vi "水样测试.vi"(11 "数据标记表":string(combo)="N") -> ()   [LabVIEW 2016, in "斯坦道多参数.lvlib"]
panel:
  out "运行状态":u16(ring) items=["空闲", "水样测试", "标样核查"]
  out "多参数运行日志":string
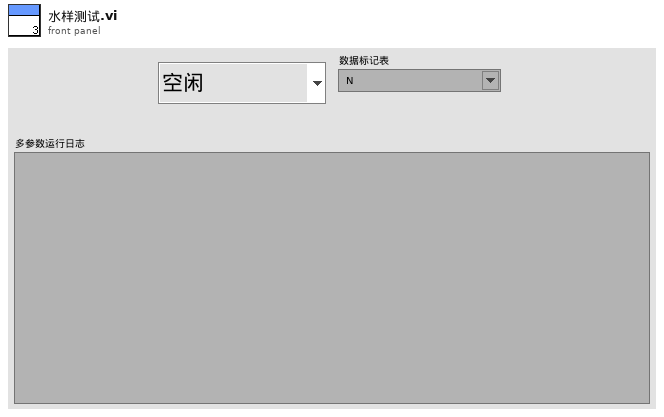
[diagram p1: front panel]
types:
  T1 = typedef "集成多参数单参数字段定义.ctl" = cluster{"时间":timestamp, "测量模式":string, "数据类型":string, "检测值":sgl, "单位":string, "数据标识":string, "信号值":sgl, "标样参考值":sgl, "因子编码":string, "探头温度":sgl, "LastTime":timestamp}
  T2 = cluster{"水温":bool, "pH":bool, "DO":bool, "DOper":bool, "电导率":bool, "ORP":bool, "浊度":bool, "叶绿素a":bool, "藻密度":bool, "COD":bool, "DO2":bool, "DOper":bool}
  T3 = cluster{"水样数据时间":timestamp, "水温":dbl, "pH":dbl, "DO":dbl, "DOper":dbl, "电导率":dbl, "ORP":dbl, "浊度":dbl, "叶绿素a":dbl, "藻密度":dbl, "COD":dbl, "DO2":dbl, "DO2per":dbl}
  T4 = cluster{"ph":bool, "DO":bool, "Cond":bool, "Turb":bool, "叶绿素a":bool, "藻密度":bool, "ORP":bool, "cod":bool, "DO2":bool}
  T5 = cluster{"温度测量值":sgl, "测量值":sgl, "温度偏移修正值":sgl, "信号值":sgl, "数据标识":string}
  T6 = cluster{"CH":u16, "监测值":dbl, "信号值":sgl, "数据标识":string}
  T7 = cluster{"温度测量值":sgl, "DO%":sgl, "DOmg/L":sgl, "温度偏移修正值":sgl, "数据标识mg/L":string, "数据标识%":string}
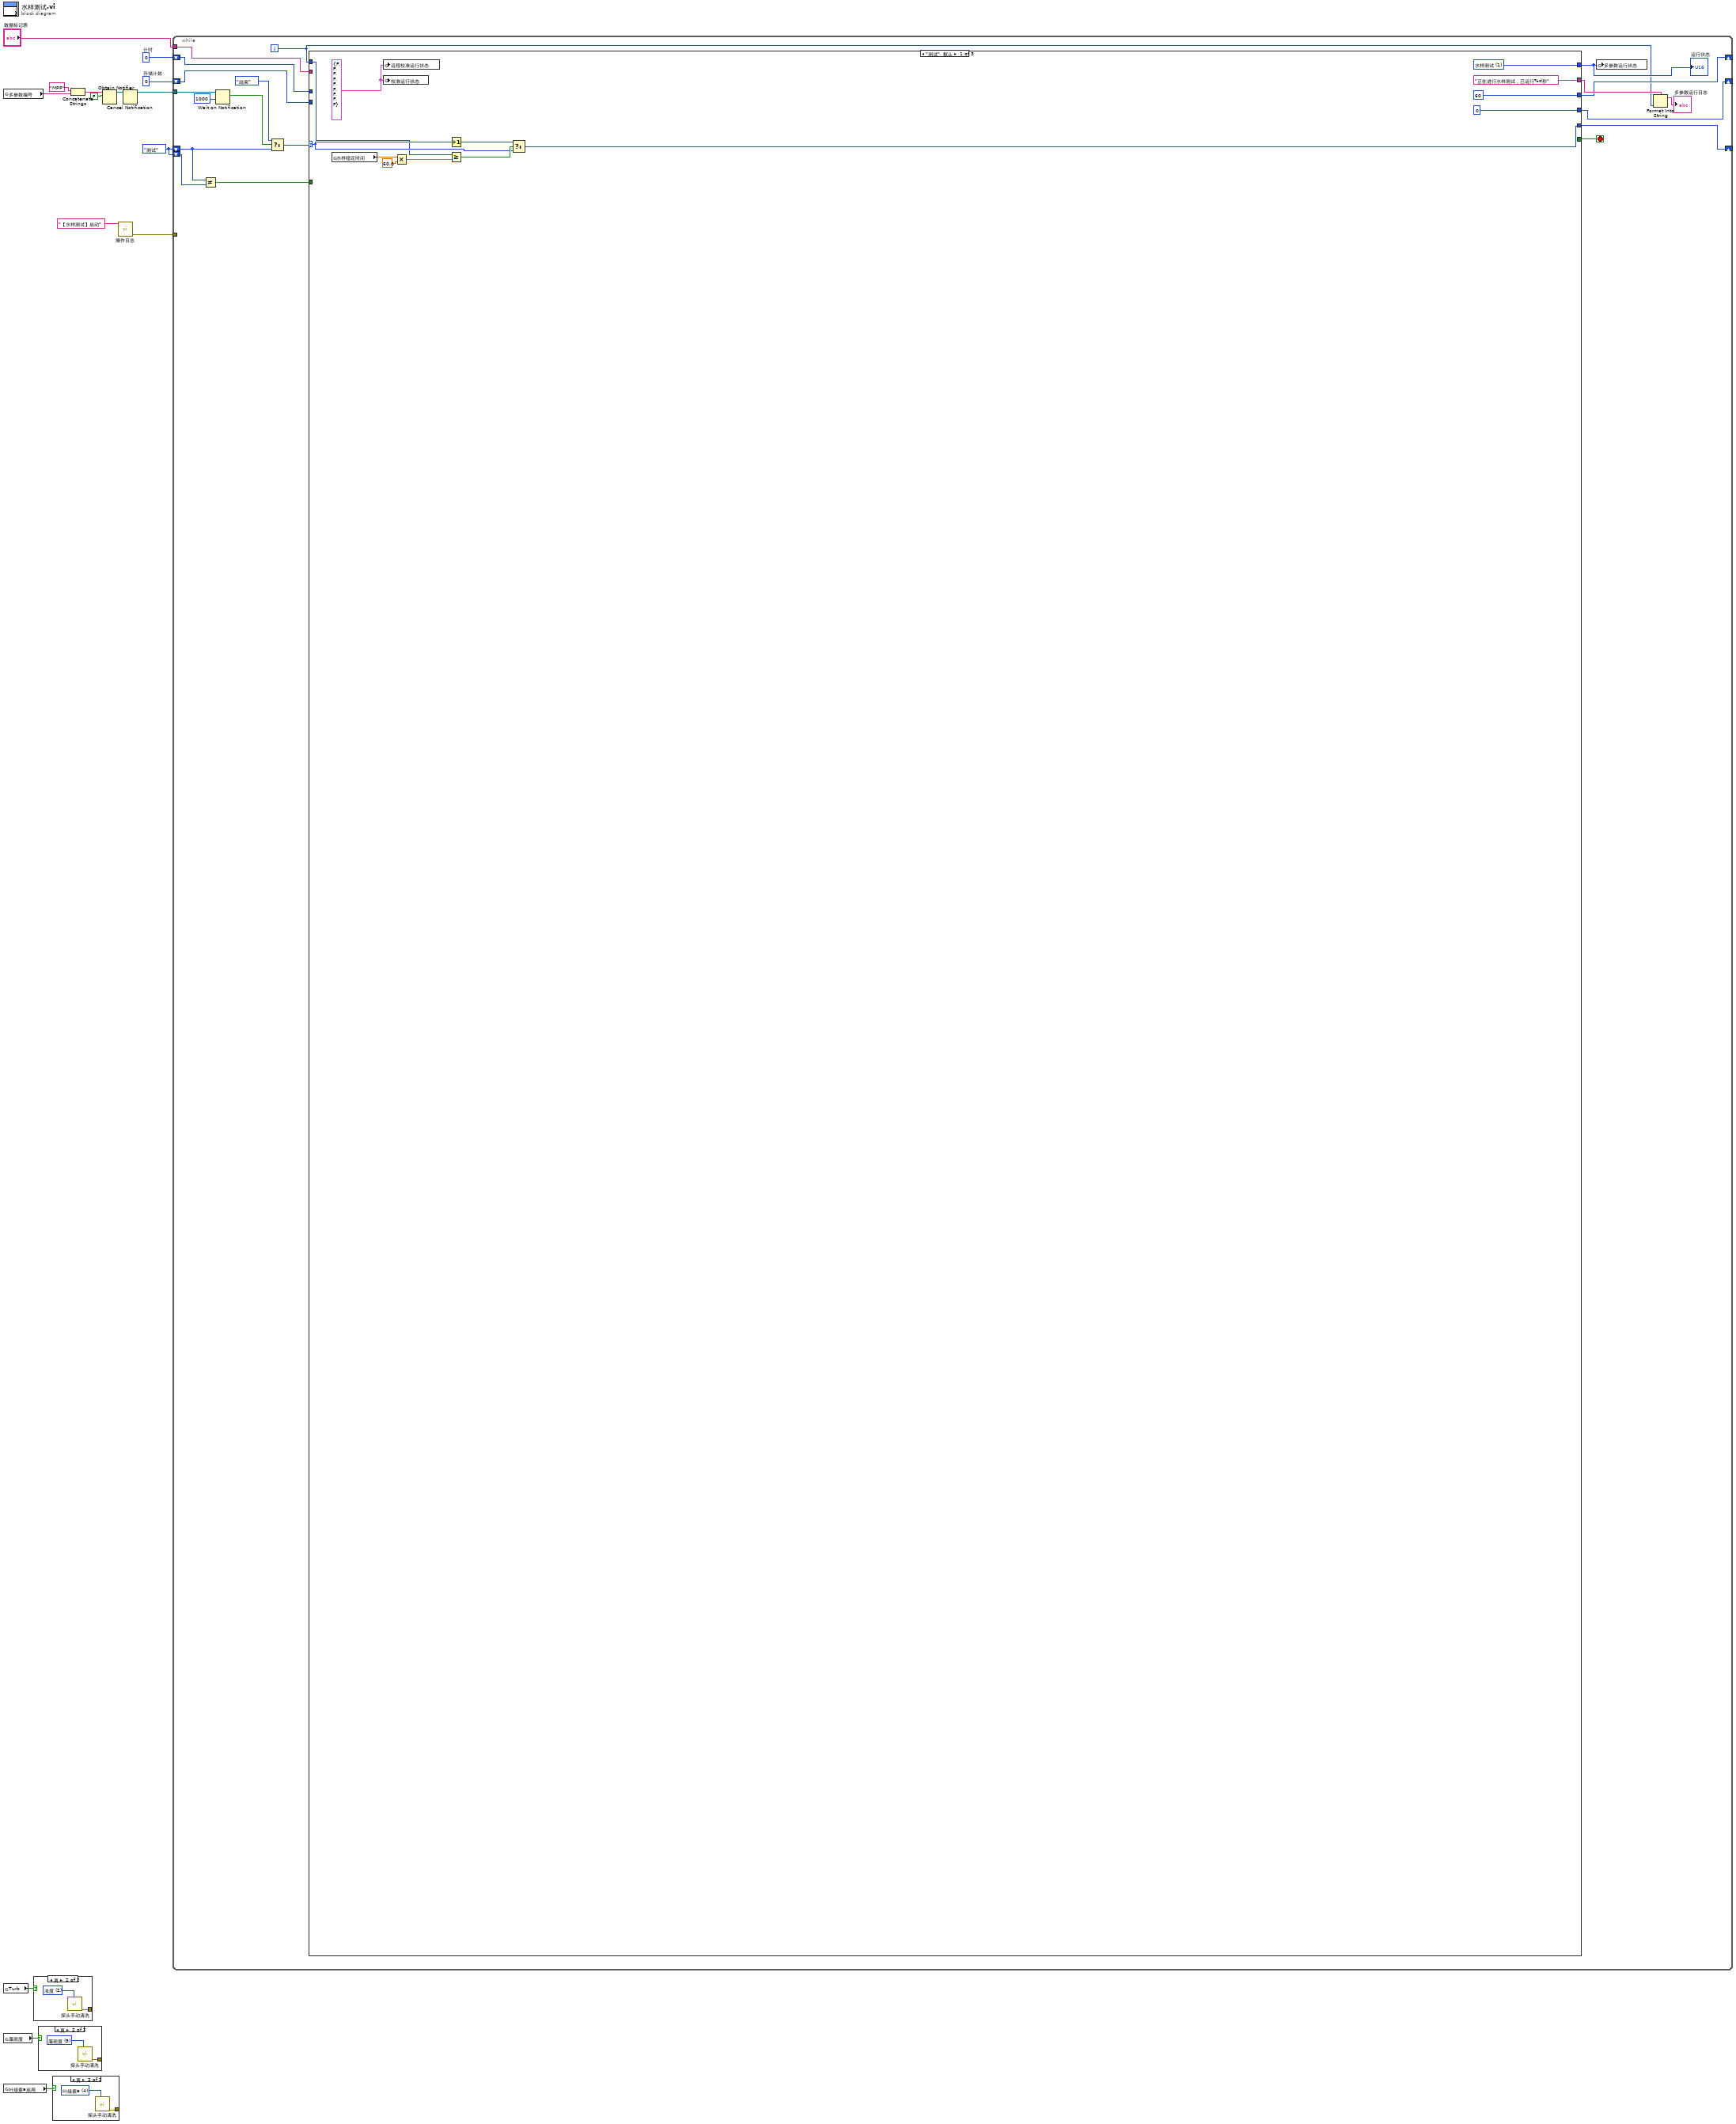
[diagram p0: block diagram]
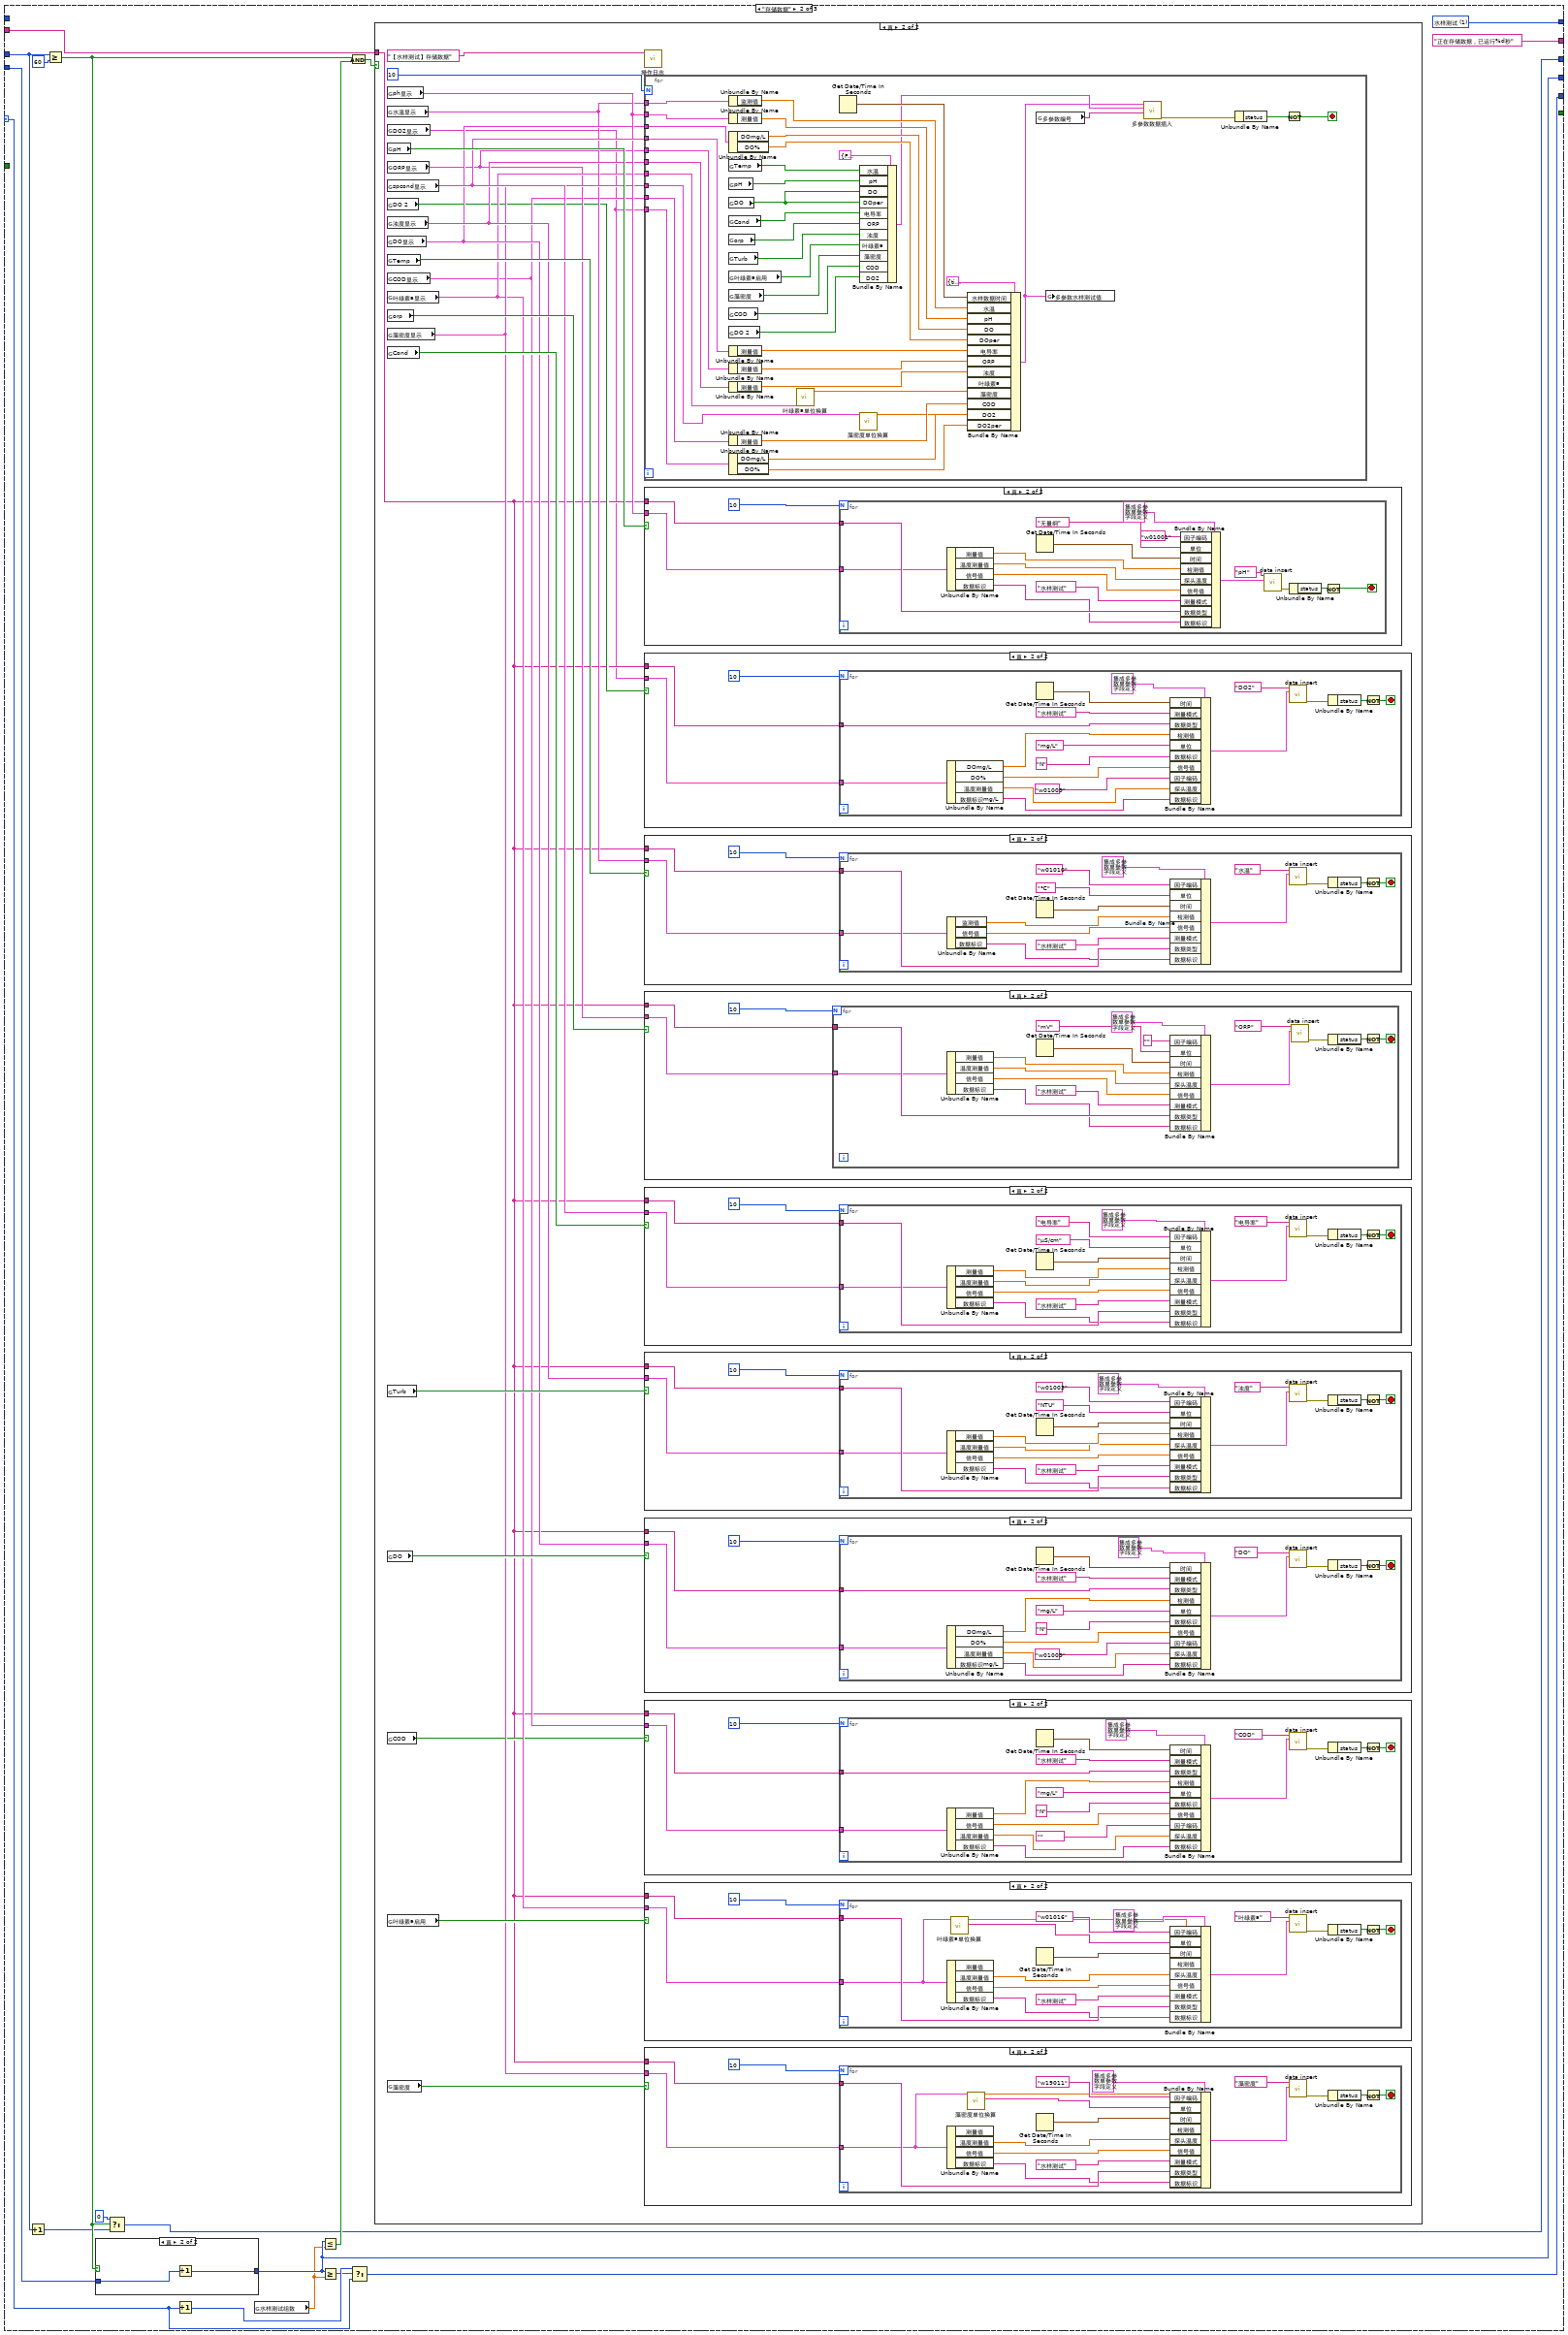
[diagram p5: hidden frame]
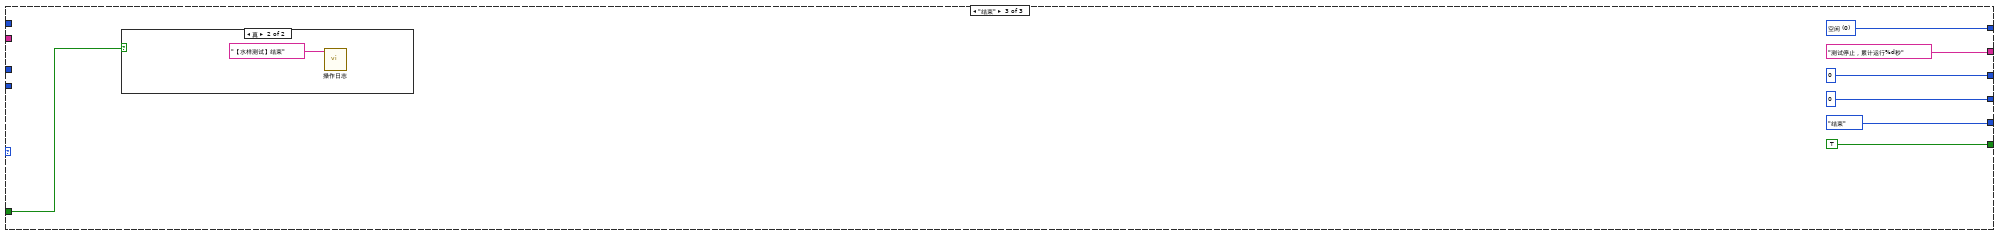
[diagram p18: hidden frame]
diagram:
  w7 = 0  # 存储计数
  w8 = 0  # 计时
  w3 = enum16{"测试", "存储数据", "结束"}."测试" ("枚举")
  n1 = global read "多参数全局变量.vi" "多参数编号"() -> (w9:string)
  n2 = global read "断电保存变量.vi" "Turb"() -> (w6:bool)
  n3 = global read "断电保存变量.vi" "藻密度"() -> (w4:bool)
  n4 = global read "断电保存变量.vi" "叶绿素a启用"() -> (w5:bool)
  n5 = case shown="真" w6 {
    tunnel: [_ w16] -> _
    frame False {
    }
    frame True {
      w17 = u16 2 items=["pH", "DO", "浊度", "电导率", "叶绿素a", "藻密度", "ORP", "DO2"] ("校准参数")
      n6 = call "探头手动清洗.vi"("校准参数"=w17) -> ("error out"=w16:errorcluster)  [unwired: 10 in]
    }
  }
  n7 = case shown="真" w4 {
    tunnel: [_ w18] -> _
    frame False {
    }
    frame True {
      w19 = u16 5 items=["pH", "DO", "浊度", "电导率", "叶绿素a", "藻密度", "ORP", "DO2"] ("校准参数")
      n8 = call "探头手动清洗.vi"("校准参数"=w19) -> ("error out"=w18:errorcluster)  [unwired: 10 in]
    }
  }
  n9 = case shown="真" w5 {
    tunnel: [_ w20] -> _
    frame False {
    }
    frame True {
      w21 = u16 4 items=["pH", "DO", "浊度", "电导率", "叶绿素a", "藻密度", "ORP", "DO2"] ("校准参数")
      n10 = call "探头手动清洗.vi"("校准参数"=w21) -> ("error out"=w20:errorcluster)  [unwired: 10 in]
    }
  }
  n11 = Concatenate Strings("MPP" ("名称（未命名）"), w9) -> (w10:string)
  n12 = Obtain Notifier(name (unnamed)=w10, notification data type=FALSE) -> (notifier out=w13:refnum<notifier>)  [unwired: 2 in, 2 out]
  n13 = call "操作日志.vi"("日志信息"="【水样测试】启动") -> ("error out"=w1:errorcluster)  [unwired: 10 in]
  n14 = Cancel Notification(0:w13) -> (8:w12:refnum<notifier>)  [unwired: 1 in, 2 out]
  n15 = while {
    shift-right: [w26] -> _
    shift-left: w3 -> [w24]
    tunnel: w12 -> [w37]
    tunnel: "数据标记表" -> [w32]
    shift-right: [w28] -> _
    shift-left: w8 -> [w30]
    shift-right: [w27] -> _
    shift-left: w7 -> [w29]
    shift-left: w3 -> [w23]
    tunnel: w1 -> [_]
    i -> [w25]
    stop <- w40 stop-if-true
    n16 = Not Equal?(x=w24, y=w23) -> (x != y?=w22:bool)
    n17 = Wait on Notification(notifier=w37, timeout in ms (-1)=1000 ("超时毫秒(-1)")) -> (notification=w35:bool)  [unwired: 2 in, 3 out]
    n18 = Select(t=enum16{"测试", "存储数据", "结束"}."结束" ("枚举"), s=w35, f=w24) -> (s? t:f=w33:enum16{"测试", "存储数据", "结束"})
    n19 = case shown="\"测试\", 默认" w33 {
      selector: w33 -> [w47 w61 _]
      tunnel: [_ _ TRUE] -> w40
      tunnel: ["正在进行水样测试，已运行%d秒" ("格式字符串") "正在存储数据，已运行%d秒" ("格式字符串") "测试停止，累计运行%d秒" ("格式字符串")] -> w39
      tunnel: [w52 w66 w335] -> w31
      tunnel: w32 -> [_ w71 _]
      tunnel: w30 -> [_ w69 _]
      tunnel: w29 -> [_ w70 _]
      tunnel: [60 w54 0] -> w28
      tunnel: [0 w60 0] -> w27
      tunnel: [w45 w64 enum16{"测试", "存储数据", "结束"}."结束" ("枚举")] -> w26
      tunnel: w25 -> [w41 _ _]
      tunnel: w22 -> [_ _ w331]
      frame "测试", Default {
        w42 = T4 {"ph"=FALSE, "DO"=FALSE, "Cond"=FALSE, "Turb"=FALSE, "叶绿素a"=FALSE, "藻密度"=FALSE, "ORP"=FALSE, "cod"=FALSE, "DO2"=FALSE} ("远程校准运行状态")
        w52 = u16 1 items=["空闲", "水样测试", "标样核查"] ("多参数运行状态")
        n20 = global read "断电保存变量.vi" "水样稳定时间"() -> (w51:dbl)
        n21 = global write "多参数全局变量.vi" "远程校准运行状态"(w42) -> ()
        n22 = global write "多参数全局变量.vi" "校准运行状态"(w42) -> ()
        n23 = Multiply(x=w51, y=60.0) -> (x*y=w49:dbl)
        n24 = Increment(x=w47) -> (x+1=w46:enum16{"测试", "存储数据", "结束"})
        n25 = Greater Or Equal?(x=w41, y=w49) -> (x >= y?=w48:bool)
        n26 = Select(t=w46, s=w48, f=w47) -> (s? t:f=w45:enum16{"测试", "存储数据", "结束"})
      }
      frame "存储数据" {
        w66 = u16 1 items=["空闲", "水样测试", "标样核查"] ("多参数运行状态")
        n27 = Increment(x=w69) -> (x+1=w56:i32)
        n28 = Greater Or Equal?(x=w69, y=60) -> (x >= y?=w57:bool)
        n29 = case shown="真" w57 {
          tunnel: w70 -> [w72 w74]
          tunnel: [w72 w73] -> w60
          frame False {
          }
          frame True {
            n30 = Increment(x=w74) -> (x+1=w73:i32)
          }
        }
        n31 = Select(t=0, s=w57, f=w56) -> (s? t:f=w54:i32)
        n32 = Increment(x=w61) -> (x+1=w62:enum16{"测试", "存储数据", "结束"})
        n33 = global read "断电保存变量.vi" "水样测试组数"() -> (w59:dbl)
        n34 = Less Or Equal?(x=w60, y=w59) -> (x <= y?=w65:bool)
        n35 = Greater Or Equal?(x=w60, y=w59) -> (x >= y?=w58:bool)
        n36 = And(x=w57, y=w65) -> (x .and. y?=w63:bool)
        n37 = Select(t=w62, s=w58, f=w61) -> (s? t:f=w64:enum16{"测试", "存储数据", "结束"})
        n38 = case shown="真" w63 {
          tunnel: w71 -> [_ w76]
          frame False {
          }
          frame True {
            n39 = global read "多参数全局变量.vi" "ph显示"() -> (w87:T5)
            n40 = global read "多参数全局变量.vi" "水温显示"() -> (w83:T6)
            n41 = global read "多参数全局变量.vi" "DO2显示"() -> (w75:T7)
            n42 = global read "断电保存变量.vi" "pH"() -> (w93:bool)
            n43 = global read "多参数全局变量.vi" "ORP显示"() -> (w81:T5)
            n44 = global read "多参数全局变量.vi" "spcond显示"() -> (w88:T5)
            n45 = global read "断电保存变量.vi" "DO 2"() -> (w77:bool)
            n46 = global read "多参数全局变量.vi" "浊度显示"() -> (w86:T5)
            n47 = global read "多参数全局变量.vi" "DO显示"() -> (w85:T7)
            n48 = global read "断电保存变量.vi" "Temp"() -> (w92:bool)
            n49 = global read "多参数全局变量.vi" "COD显示"() -> (w79:T5)
            n50 = global read "多参数全局变量.vi" "叶绿素a显示"() -> (w82:T5)
            n51 = global read "断电保存变量.vi" "orp"() -> (w90:bool)
            n52 = global read "多参数全局变量.vi" "藻密度显示"() -> (w84:T5)
            n53 = global read "断电保存变量.vi" "Cond"() -> (w95:bool)
            n54 = global read "断电保存变量.vi" "Turb"() -> (w96:bool)
            n55 = global read "断电保存变量.vi" "DO"() -> (w94:bool)
            n56 = global read "断电保存变量.vi" "COD"() -> (w78:bool)
            n57 = global read "断电保存变量.vi" "叶绿素a启用"() -> (w97:bool)
            n58 = global read "断电保存变量.vi" "藻密度"() -> (w91:bool)
            n59 = call "操作日志.vi"("日志信息"="【水样测试】存储数据") -> ()  [unwired: 10 in, 1 out]
            n60 = for {
              N: 10 -> [_]
              tunnel: w83 -> [w158]
              tunnel: w87 -> [w157]
              tunnel: w85 -> [w156]
              tunnel: w88 -> [w155]
              tunnel: w81 -> [w154]
              tunnel: w86 -> [w153]
              tunnel: w82 -> [w139]
              tunnel: w84 -> [w141]
              tunnel: w79 -> [w151]
              tunnel: w75 -> [w147]
              stop <- w160 stop-if-true
              n61 = Unbundle By Name(w158) -> ("监测值"=w177:dbl)
              n62 = Unbundle By Name(w157) -> ("测量值"=w176:sgl)
              n63 = Unbundle By Name(w156) -> ("DOmg/L"=w175:sgl, "DO%"=w174:sgl)
              n64 = global read "断电保存变量.vi" "Temp"() -> (w166:bool)
              n65 = global read "断电保存变量.vi" "pH"() -> (w170:bool)
              n66 = global read "断电保存变量.vi" "DO"() -> (w163:bool)
              n67 = global read "断电保存变量.vi" "Cond"() -> (w169:bool)
              n68 = global read "断电保存变量.vi" "orp"() -> (w165:bool)
              n69 = global read "断电保存变量.vi" "Turb"() -> (w168:bool)
              n70 = global read "断电保存变量.vi" "叶绿素a启用"() -> (w164:bool)
              n71 = global read "断电保存变量.vi" "藻密度"() -> (w167:bool)
              n72 = global read "断电保存变量.vi" "COD"() -> (w152:bool)
              n73 = global read "断电保存变量.vi" "DO 2"() -> (w148:bool)
              n74 = Unbundle By Name(w155) -> ("测量值"=w173:sgl)
              n75 = Unbundle By Name(w154) -> ("测量值"=w172:sgl)
              n76 = Unbundle By Name(w153) -> ("测量值"=w171:sgl)
              n77 = Unbundle By Name(w151) -> ("测量值"=w150:sgl)
              n78 = Unbundle By Name(w147) -> ("DOmg/L"=w146:sgl, "DO%"=w145:sgl)
              n79 = call "叶绿素a单位换算.vi"("叶绿素a显示"=w139) -> ("测量值"=w138:sgl)  [unwired: 8 in, 2 out]
              n80 = Get Date/Time In Seconds() -> (seconds since 1Jan1904=w178:timestamp)
              n81 = Bundle By Name(cluster=T2 {"水温"=FALSE, "pH"=FALSE, "DO"=FALSE, "DOper"=FALSE, "电导率"=FALSE, "ORP"=FALSE, "浊度"=FALSE, "叶绿素a"=FALSE, "藻密度"=FALSE, "COD"=FALSE, "DO2"=FALSE, "DOper"=FALSE} ("columns enable"), "水温"=w166, "pH"=w170, "DO"=w163, "DOper"=w163, "电导率"=w169, "ORP"=w165, "浊度"=w168, "叶绿素a"=w164, "藻密度"=w167, "COD"=w152, "DO2"=w148) -> (w143:T2)
              n82 = call "藻密度单位换算.vi"("藻密度显示"=w141) -> ("测量值"=w140:sgl)  [unwired: 8 in, 2 out]
              n83 = Bundle By Name(cluster=T3 {"水样数据时间"=timestamp(0 s since 1904-01-01), "水温"=0.0, "pH"=0.0, "DO"=0.0, "DOper"=0.0, "电导率"=0.0, "ORP"=0.0, "浊度"=0.0, "叶绿素a"=0.0, "藻密度"=0.0, "COD"=0.0, "DO2"=0.0, "DO2per"=0.0} ("data in"), "水样数据时间"=w178, "水温"=w177, "pH"=w176, "DO"=w175, "DOper"=w174, "电导率"=w173, "ORP"=w172, "浊度"=w171, "叶绿素a"=w138, "藻密度"=w140, "COD"=w150, "DO2"=w146, "DO2per"=w145) -> (w142:T3)
              n84 = global read "多参数全局变量.vi" "多参数编号"() -> (w159:string)
              n85 = global write "多参数全局变量.vi" "多参数水样测试值"(w142) -> ()
              n86 = call "多参数数据插入.vi"("编号"=w159, "columns enable"=w143, "data in"=w142) -> ("error out"=w162:errorcluster)  [unwired: 8 in]
              n87 = Unbundle By Name(w162) -> ("status"=w161:bool)
              n88 = Not(x=w161) -> (.not. x?=w160:bool)
            }
            n89 = case shown="真" w93 {
              tunnel: w76 -> [_ w296]
              tunnel: w87 -> [_ w294]
              frame False {
              }
              frame True {
                n90 = for {
                  N: 10 -> [_]
                  tunnel: w296 -> [w300]
                  tunnel: w294 -> [w299]
                  stop <- w304 stop-if-true
                  n91 = Unbundle By Name(w299) -> ("测量值"=w308:sgl, "温度测量值"=w307:sgl, "信号值"=w302:sgl, "数据标识"=w298:string)
                  n92 = Get Date/Time In Seconds() -> (seconds since 1Jan1904=w303:timestamp)
                  n93 = Bundle By Name(cluster=T1 {"时间"=timestamp(0 s since 1904-01-01), "测量模式"="水样测试", "数据类型"="N", "检测值"=0.0, "单位"="mg/L", "数据标识"="N", "信号值"=0.0, "标样参考值"=0.0, "因子编码"="", "探头温度"=0.0, "LastTime"=timestamp(0 s since 1904-01-01)} ("data"), "因子编码"="w01001", "单位"="无量纲", "时间"=w303, "检测值"=w308, "探头温度"=w307, "信号值"=w302, "测量模式"="水样测试", "数据类型"=w300, "数据标识"=w298) -> (w312:T1)
                  n94 = call "data insert.vi"("data"=w312, "table in"="pH" ("table输入")) -> ("error out"=w306:errorcluster)  [unwired: 9 in]
                  n95 = Unbundle By Name(w306) -> ("status"=w305:bool)
                  n96 = Not(x=w305) -> (.not. x?=w304:bool)
                }
              }
            }
            n97 = case shown="真" w77 {
              tunnel: w76 -> [_ w100]
              tunnel: w75 -> [_ w98]
              frame False {
              }
              frame True {
                n98 = for {
                  N: 10 -> [_]
                  tunnel: w100 -> [w114]
                  tunnel: w98 -> [w104]
                  stop <- w117 stop-if-true
                  n99 = Unbundle By Name(w104) -> ("DOmg/L"=w113:sgl, "DO%"=w106:sgl, "温度测量值"=w107:sgl, "数据标识mg/L"=w103:string)
                  n100 = Get Date/Time In Seconds() -> (seconds since 1Jan1904=w116:timestamp)
                  n101 = Bundle By Name(cluster=T1 {"时间"=timestamp(0 s since 1904-01-01), "测量模式"="水样测试", "数据类型"="N", "检测值"=0.0, "单位"="mg/L", "数据标识"="N", "信号值"=0.0, "标样参考值"=0.0, "因子编码"="", "探头温度"=0.0, "LastTime"=timestamp(0 s since 1904-01-01)} ("data"), "时间"=w116, "测量模式"="水样测试", "数据类型"=w114, "检测值"=w113, "单位"="mg/L", "数据标识"="N" ("水样数据标识"), "信号值"=w106, "因子编码"="w01009", "探头温度"=w107, "数据标识"=w103) -> (w105:T1)
                  n102 = call "data insert.vi"("data"=w105, "table in"="DO2") -> ("error out"=w109:errorcluster)  [unwired: 9 in]
                  n103 = Unbundle By Name(w109) -> ("status"=w110:bool)
                  n104 = Not(x=w110) -> (.not. x?=w117:bool)
                }
              }
            }
            n105 = case shown="真" w92 {
              tunnel: w76 -> [_ w315]
              tunnel: w83 -> [_ w313]
              frame False {
              }
              frame True {
                n106 = for {
                  N: 10 -> [_]
                  tunnel: w315 -> [w319]
                  tunnel: w313 -> [w318]
                  stop <- w323 stop-if-true
                  n107 = Unbundle By Name(w318) -> ("监测值"=w326:dbl, "信号值"=w321:sgl, "数据标识"=w317:string)
                  n108 = Get Date/Time In Seconds() -> (seconds since 1Jan1904=w322:timestamp)
                  n109 = Bundle By Name(cluster=T1 {"时间"=timestamp(0 s since 1904-01-01), "测量模式"="水样测试", "数据类型"="N", "检测值"=0.0, "单位"="mg/L", "数据标识"="N", "信号值"=0.0, "标样参考值"=0.0, "因子编码"="", "探头温度"=0.0, "LastTime"=timestamp(0 s since 1904-01-01)} ("data"), "因子编码"="w01010", "单位"="℃", "时间"=w322, "检测值"=w326, "信号值"=w321, "测量模式"="水样测试", "数据类型"=w319, "数据标识"=w317) -> (w329:T1)
                  n110 = call "data insert.vi"("data"=w329, "table in"="水温" ("table输入")) -> ("error out"=w325:errorcluster)  [unwired: 9 in]
                  n111 = Unbundle By Name(w325) -> ("status"=w324:bool)
                  n112 = Not(x=w324) -> (.not. x?=w323:bool)
                }
              }
            }
            n113 = case shown="真" w90 {
              tunnel: w76 -> [_ w181]
              tunnel: w81 -> [_ w179]
              frame False {
              }
              frame True {
                n114 = for {
                  N: 10 -> [_]
                  tunnel: w181 -> [w187]
                  tunnel: w179 -> [w185]
                  stop <- w190 stop-if-true
                  n115 = Unbundle By Name(w185) -> ("测量值"=w197:sgl, "温度测量值"=w195:sgl, "信号值"=w188:sgl, "数据标识"=w184:string)
                  n116 = Get Date/Time In Seconds() -> (seconds since 1Jan1904=w189:timestamp)
                  n117 = Bundle By Name(cluster=T1 {"时间"=timestamp(0 s since 1904-01-01), "测量模式"="水样测试", "数据类型"="N", "检测值"=0.0, "单位"="mg/L", "数据标识"="N", "信号值"=0.0, "标样参考值"=0.0, "因子编码"="", "探头温度"=0.0, "LastTime"=timestamp(0 s since 1904-01-01)} ("data"), "因子编码"="", "单位"="mV", "时间"=w189, "检测值"=w197, "探头温度"=w195, "信号值"=w188, "测量模式"="水样测试", "数据类型"=w187, "数据标识"=w184) -> (w182:T1)
                  n118 = call "data insert.vi"("data"=w182, "table in"="ORP" ("table输入")) -> ("error out"=w193:errorcluster)  [unwired: 9 in]
                  n119 = Unbundle By Name(w193) -> ("status"=w192:bool)
                  n120 = Not(x=w192) -> (.not. x?=w190:bool)
                }
              }
            }
            n121 = case shown="真" w95 {
              tunnel: w76 -> [_ w257]
              tunnel: w88 -> [_ w255]
              frame False {
              }
              frame True {
                n122 = for {
                  N: 10 -> [_]
                  tunnel: w257 -> [w261]
                  tunnel: w255 -> [w260]
                  stop <- w266 stop-if-true
                  n123 = Unbundle By Name(w260) -> ("测量值"=w271:sgl, "温度测量值"=w270:sgl, "信号值"=w264:sgl, "数据标识"=w259:string)
                  n124 = Get Date/Time In Seconds() -> (seconds since 1Jan1904=w265:timestamp)
                  n125 = Bundle By Name(cluster=T1 {"时间"=timestamp(0 s since 1904-01-01), "测量模式"="水样测试", "数据类型"="N", "检测值"=0.0, "单位"="mg/L", "数据标识"="N", "信号值"=0.0, "标样参考值"=0.0, "因子编码"="", "探头温度"=0.0, "LastTime"=timestamp(0 s since 1904-01-01)} ("data"), "因子编码"="电导率", "单位"="μS/cm", "时间"=w265, "检测值"=w271, "探头温度"=w270, "信号值"=w264, "测量模式"="水样测试", "数据类型"=w261, "数据标识"=w259) -> (w262:T1)
                  n126 = call "data insert.vi"("data"=w262, "table in"="电导率" ("table输入")) -> ("error out"=w269:errorcluster)  [unwired: 9 in]
                  n127 = Unbundle By Name(w269) -> ("status"=w268:bool)
                  n128 = Not(x=w268) -> (.not. x?=w266:bool)
                }
              }
            }
            n129 = case shown="真" w96 {
              tunnel: w76 -> [_ w238]
              tunnel: w86 -> [_ w236]
              frame False {
              }
              frame True {
                n130 = for {
                  N: 10 -> [_]
                  tunnel: w238 -> [w242]
                  tunnel: w236 -> [w241]
                  stop <- w246 stop-if-true
                  n131 = Unbundle By Name(w241) -> ("测量值"=w250:sgl, "温度测量值"=w249:sgl, "信号值"=w244:sgl, "数据标识"=w240:string)
                  n132 = Get Date/Time In Seconds() -> (seconds since 1Jan1904=w245:timestamp)
                  n133 = Bundle By Name(cluster=T1 {"时间"=timestamp(0 s since 1904-01-01), "测量模式"="水样测试", "数据类型"="N", "检测值"=0.0, "单位"="mg/L", "数据标识"="N", "信号值"=0.0, "标样参考值"=0.0, "因子编码"="", "探头温度"=0.0, "LastTime"=timestamp(0 s since 1904-01-01)} ("data"), "因子编码"="w01003", "单位"="NTU", "时间"=w245, "检测值"=w250, "探头温度"=w249, "信号值"=w244, "测量模式"="水样测试", "数据类型"=w242, "数据标识"=w240) -> (w253:T1)
                  n134 = call "data insert.vi"("data"=w253, "table in"="浊度" ("table输入")) -> ("error out"=w248:errorcluster)  [unwired: 9 in]
                  n135 = Unbundle By Name(w248) -> ("status"=w247:bool)
                  n136 = Not(x=w247) -> (.not. x?=w246:bool)
                }
              }
            }
            n137 = case shown="真" w94 {
              tunnel: w76 -> [_ w276]
              tunnel: w85 -> [_ w274]
              frame False {
              }
              frame True {
                n138 = for {
                  N: 10 -> [_]
                  tunnel: w276 -> [w289]
                  tunnel: w274 -> [w279]
                  stop <- w293 stop-if-true
                  n139 = Unbundle By Name(w279) -> ("DOmg/L"=w288:sgl, "DO%"=w281:sgl, "温度测量值"=w282:sgl, "数据标识mg/L"=w278:string)
                  n140 = Get Date/Time In Seconds() -> (seconds since 1Jan1904=w291:timestamp)
                  n141 = Bundle By Name(cluster=T1 {"时间"=timestamp(0 s since 1904-01-01), "测量模式"="水样测试", "数据类型"="N", "检测值"=0.0, "单位"="mg/L", "数据标识"="N", "信号值"=0.0, "标样参考值"=0.0, "因子编码"="", "探头温度"=0.0, "LastTime"=timestamp(0 s since 1904-01-01)} ("data"), "时间"=w291, "测量模式"="水样测试", "数据类型"=w289, "检测值"=w288, "单位"="mg/L", "数据标识"="N" ("水样数据标识"), "信号值"=w281, "因子编码"="w01009", "探头温度"=w282, "数据标识"=w278) -> (w280:T1)
                  n142 = call "data insert.vi"("data"=w280, "table in"="DO") -> ("error out"=w284:errorcluster)  [unwired: 9 in]
                  n143 = Unbundle By Name(w284) -> ("status"=w285:bool)
                  n144 = Not(x=w285) -> (.not. x?=w293:bool)
                }
              }
            }
            n145 = case shown="真" w78 {
              tunnel: w76 -> [_ w120]
              tunnel: w79 -> [_ w118]
              frame False {
              }
              frame True {
                n146 = for {
                  N: 10 -> [_]
                  tunnel: w120 -> [w133]
                  tunnel: w118 -> [w123]
                  stop <- w137 stop-if-true
                  n147 = Unbundle By Name(w123) -> ("测量值"=w132:sgl, "信号值"=w125:sgl, "温度测量值"=w126:sgl, "数据标识"=w122:string)
                  n148 = Get Date/Time In Seconds() -> (seconds since 1Jan1904=w135:timestamp)
                  n149 = Bundle By Name(cluster=T1 {"时间"=timestamp(0 s since 1904-01-01), "测量模式"="水样测试", "数据类型"="N", "检测值"=0.0, "单位"="mg/L", "数据标识"="N", "信号值"=0.0, "标样参考值"=0.0, "因子编码"="", "探头温度"=0.0, "LastTime"=timestamp(0 s since 1904-01-01)} ("data"), "时间"=w135, "测量模式"="水样测试", "数据类型"=w133, "检测值"=w132, "单位"="mg/L", "数据标识"="N" ("水样数据标识"), "信号值"=w125, "因子编码"="", "探头温度"=w126, "数据标识"=w122) -> (w124:T1)
                  n150 = call "data insert.vi"("data"=w124, "table in"="COD") -> ("error out"=w128:errorcluster)  [unwired: 9 in]
                  n151 = Unbundle By Name(w128) -> ("status"=w129:bool)
                  n152 = Not(x=w129) -> (.not. x?=w137:bool)
                }
              }
            }
            n153 = case shown="真" w97 {
              tunnel: w76 -> [_ w219]
              tunnel: w82 -> [_ w217]
              frame False {
              }
              frame True {
                n154 = for {
                  N: 10 -> [_]
                  tunnel: w219 -> [w225]
                  tunnel: w217 -> [w222]
                  stop <- w229 stop-if-true
                  n155 = Unbundle By Name(w222) -> ("温度测量值"=w235:sgl, "信号值"=w228:sgl, "数据标识"=w224:string)  [unwired: 1 out]
                  n156 = call "叶绿素a单位换算.vi"("叶绿素a显示"=w222) -> ("检测值1.单位"=w221:string, "测量值"=w220:sgl)  [unwired: 8 in, 1 out]
                  n157 = Get Date/Time In Seconds() -> (seconds since 1Jan1904=w227:timestamp)
                  n158 = Bundle By Name(cluster=T1 {"时间"=timestamp(0 s since 1904-01-01), "测量模式"="水样测试", "数据类型"="N", "检测值"=0.0, "单位"="mg/L", "数据标识"="N", "信号值"=0.0, "标样参考值"=0.0, "因子编码"="", "探头温度"=0.0, "LastTime"=timestamp(0 s since 1904-01-01)} ("data"), "因子编码"="w01016", "单位"=w221, "时间"=w227, "检测值"=w220, "探头温度"=w235, "信号值"=w228, "测量模式"="水样测试", "数据类型"=w225, "数据标识"=w224) -> (w233:T1)
                  n159 = call "data insert.vi"("data"=w233, "table in"="叶绿素a" ("table输入")) -> ("error out"=w231:errorcluster)  [unwired: 9 in]
                  n160 = Unbundle By Name(w231) -> ("status"=w230:bool)
                  n161 = Not(x=w230) -> (.not. x?=w229:bool)
                }
              }
            }
            n162 = case shown="真" w91 {
              tunnel: w76 -> [_ w200]
              tunnel: w84 -> [_ w198]
              frame False {
              }
              frame True {
                n163 = for {
                  N: 10 -> [_]
                  tunnel: w200 -> [w207]
                  tunnel: w198 -> [w203]
                  stop <- w208 stop-if-true
                  n164 = Unbundle By Name(w203) -> ("温度测量值"=w216:sgl, "信号值"=w209:sgl, "数据标识"=w205:string)  [unwired: 1 out]
                  n165 = call "藻密度单位换算.vi"("藻密度显示"=w203) -> ("检测值1.单位"=w201:string, "测量值"=w202:sgl)  [unwired: 8 in, 1 out]
                  n166 = Get Date/Time In Seconds() -> (seconds since 1Jan1904=w210:timestamp)
                  n167 = Bundle By Name(cluster=T1 {"时间"=timestamp(0 s since 1904-01-01), "测量模式"="水样测试", "数据类型"="N", "检测值"=0.0, "单位"="mg/L", "数据标识"="N", "信号值"=0.0, "标样参考值"=0.0, "因子编码"="", "探头温度"=0.0, "LastTime"=timestamp(0 s since 1904-01-01)} ("data"), "因子编码"="w19011", "单位"=w201, "时间"=w210, "检测值"=w202, "探头温度"=w216, "信号值"=w209, "测量模式"="水样测试", "数据类型"=w207, "数据标识"=w205) -> (w211:T1)
                  n168 = call "data insert.vi"("data"=w211, "table in"="藻密度" ("table输入")) -> ("error out"=w213:errorcluster)  [unwired: 9 in]
                  n169 = Unbundle By Name(w213) -> ("status"=w212:bool)
                  n170 = Not(x=w212) -> (.not. x?=w208:bool)
                }
              }
            }
          }
        }
      }
      frame "结束" {
        w335 = u16 0 items=["空闲", "水样测试", "标样核查"] ("多参数运行状态")
        n171 = case shown="真" w331 {
          frame False {
          }
          frame True {
            n172 = call "操作日志.vi"("日志信息"="【水样测试】结束") -> ()  [unwired: 10 in, 1 out]
          }
        }
      }
    }
    "运行状态" <- w31
    n173 = global write "多参数全局变量.vi" "多参数运行状态"(w31) -> ()
    n174 = Format Into String(format string=w39, w25) -> (resulting string=→"多参数运行日志":string)  [unwired: 2 in, 1 out]
  }
